vi "New Child.vi"(7 "Value Type (Object)":T1=enum."Object", 8 "error in (no error)":errorcluster, 10 "Child Name":string, 11 "Config Element in":refnum<class "Config Element.lvclass">) -> (0 "error out":errorcluster, 2 "New Child":refnum<class "Config Element.lvclass">, 3 "Config Element out":refnum<class "Config Element.lvclass">)   [LabVIEW 2023, in "CDM-Config.lvlib" / "Config Element.lvclass"]
doc: "Creates a new direct child under this element. The new child will not have a value or any meta values set on it."
uses:
  Config Element.lvclass
  Value Type.ctl
  Config Element.lvclass/Config Element.ctl
  <vilib>/Utility/error.llb/Error Cluster From Error Code.vi
  Config Manager/Config Manager.lvclass
  CDM-Config.lvlib
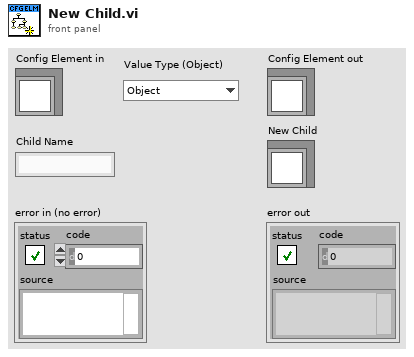
[diagram p1: front panel]
types:
  T1 = typedef "CDM-Config.lvlib/Value Type.ctl" = enum16{"String", "Number", "Bool", "Object", "Array"}
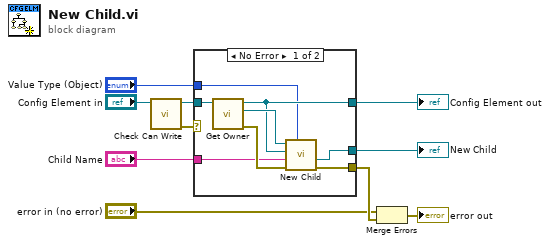
[diagram p0: block diagram]
diagram:
  n1 = call "Check Can Write.vi"("Config Element in"="Config Element in") -> ("error out"=w4:errorcluster, "Config Element out"=w5:refnum<class "Config Element.lvclass">)  [unwired: 9 in]
  n2 = case shown="No Error" w4 {
    selector: w4 -> [_ w19]
    tunnel: w5 -> [w18 w20]
    tunnel: "Child Name" -> [w15 _]
    tunnel: [w14 w20] -> w8
    tunnel: [w13 _] -> w7
    tunnel: "Value Type (Object)" -> [w12 _]
    tunnel: [w11 w19] -> w3
    frame No Error {
      n3 = call "Get Owner.vi"("Config Element in"=w18) -> ("error out"=w17:errorcluster, "Owner"=w16:refnum<class "Config Manager.lvclass">, "Config Element out"=w14:refnum<class "Config Element.lvclass">)  [unwired: 8 in]
      n4 = call "New Child.vi"("Value Type (Object)"=w12, "error in (no error)"=w17, "Child Name"=w15, "Parent"=w14, "Config Manager in"=w16) -> ("error out"=w11:errorcluster, "New Child"=w13:refnum<class "Config Element.lvclass">)  [unwired: 4 in, 1 out]
    }
    frame Error {
    }
  }
  "Config Element out" <- w8
  "New Child" <- w7
  n5 = Merge Errors("error in (no error)", w3) -> (→"error out":errorcluster)
